vi "QSM - Add State(s) to Back.vi"(6 "QSM":T1={"Invalid Option"=enum."Ignore", "QSM"=refnum}, 7 "Act? (T)":bool=TRUE, 8 "error in (no error)":errorcluster, 11 "State(s)":string) -> (0 "error out":errorcluster)   [LabVIEW 2014]
doc: "This VI enqueues multiple states. To add a new state, simply type in the state in a new line.\n\nDataEtc Copyright (c) 2013"
uses:
  TypeDef/QSM - STYP.ctl
  TypeDef/Invalid Option - STYP.ctl
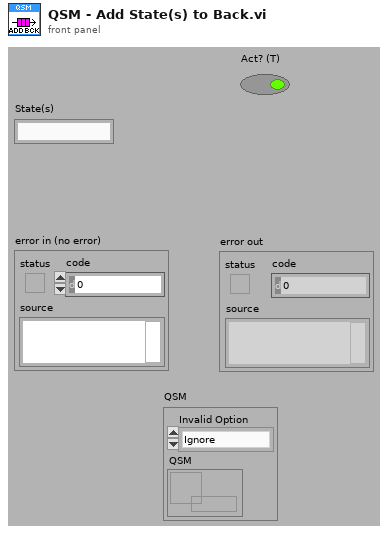
[diagram p1: front panel]
types:
  T1 = typedef "QSM - STYP.ctl" = cluster{"Invalid Option":T2, "QSM":refnum<queue>}
  T2 = typedef "Invalid Option - STYP.ctl" = enum16{"Dialog", "Error", "Ignore"}
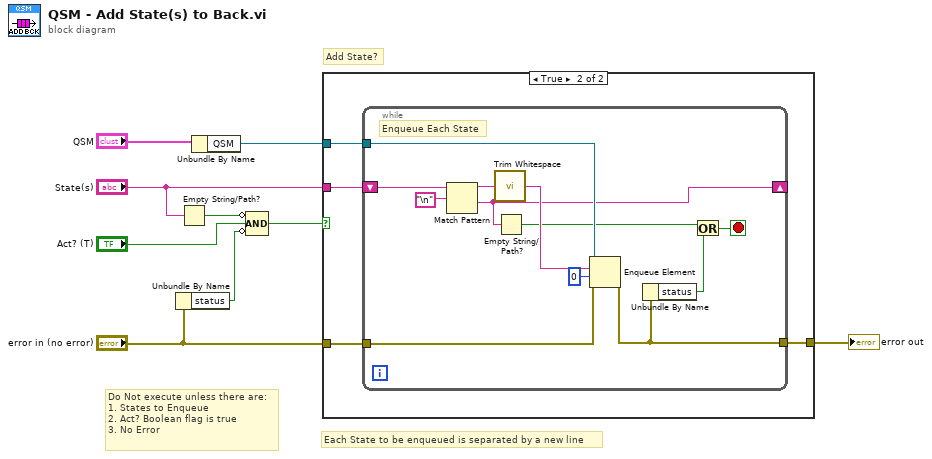
[diagram p0: block diagram]
diagram:
  # "Do Not execute unless there are:\n1. States to Enqueue\n2. Act? Boolean flag is true\n3. No Error"
  # "Each State to be enqueued is separated by a new line"
  # "Add State?"
  n1 = Unbundle By Name("error in (no error)") -> ("status"=w6:bool)
  n2 = Empty String/Path?(string/path="State(s)") -> (empty?=w8:bool)
  n3 = Unbundle By Name("QSM") -> ("QSM"=w2:refnum<queue>)
  n4 = Compound Arithmetic op=AND(invert w8, "Act? (T)", invert w6) -> (w5:bool)
  n5 = case shown="True" w5 {
    tunnel: "error in (no error)" -> [w10 w14]
    tunnel: "State(s)" -> [_ w12]
    tunnel: w2 -> [_ w13]
    tunnel: [w10 w11] -> w1
    frame False {
    }
    frame True {
      n6 = while {
        tunnel: w14 -> [w25]
        tunnel: w13 -> [w26]
        shift-right: [w19] -> _
        shift-left: w12 -> [w24]
        tunnel: [w18] -> w11
        stop <- w15 stop-if-true
        # "Enqueue Each State"
        n7 = Match Pattern(string=w24, regular expression="\n") -> (before substring=w22:string, after substring=w19:string)  [unwired: 3 out]
        n8 = call <vilib>:"Trim Whitespace.vi"("string"=w22) -> ("trimmed string"=w21:string)  [unwired: 1 in]
        n9 = Empty String/Path?(string/path=w19) -> (empty?=w17:bool)
        n10 = Enqueue Element(queue=w26, element=w21, timeout in ms (-1)=0, error in (no error)=w25) -> (error out=w18:errorcluster)  [unwired: 2 out]
        n11 = Unbundle By Name(w18) -> ("status"=w16:bool)
        n12 = Or(x=w17, y=w16) -> (x .or. y?=w15:bool)
      }
    }
  }
  "error out" <- w1
